vi "Create Queues for Logging and Transmission.vi"(8 "error in (no error)":errorcluster caption="错误输入（无错误）") -> (0 "error out":errorcluster caption="错误输出", 3 "Queues for Logging and Transmission":T1 caption="至记录与传输循环的队列")   [LabVIEW 2013]
doc: "本VI用于创建应用程序所需的所有消息队列。如应用程序需要两个以上消息队列，可右键单击上面的“消息队列”常量并选择“打开自定义类型”，将新的消息队列添加至该自定义类型，然后通过本VI进行初始化。"
uses:
  Queues for Logging and Transmission.ctl
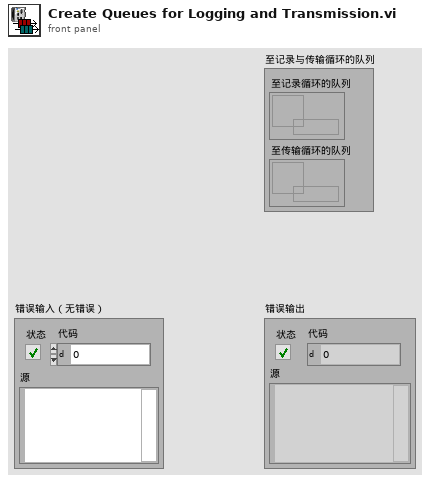
[diagram p1: front panel]
types:
  T1 = typedef "Queues for Logging and Transmission.ctl" = cluster{"Queue to Logging Loop":refnum<queue>, "Queue to Transmission Loop":refnum<queue>}
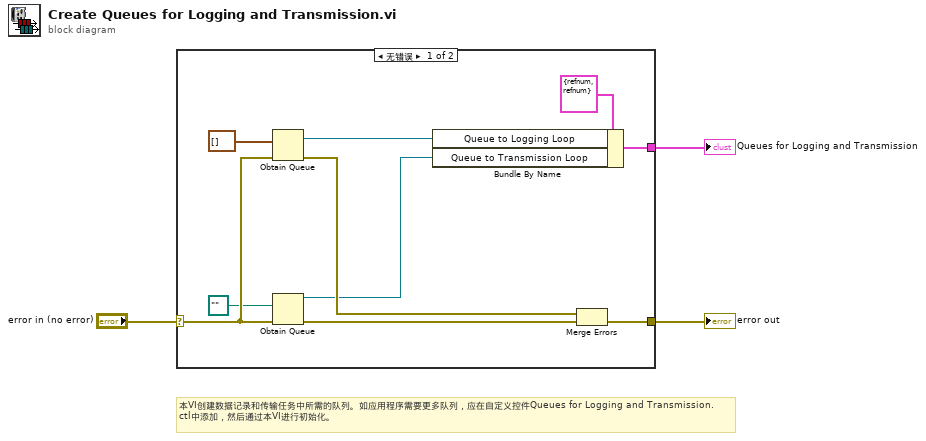
[diagram p0: block diagram]
diagram:
  # "本VI创建数据记录和传输任务中所需的队列。如应用程序需要更多队列，应在自定义控件Queues for Logging and Transmission.ctl中添加，然后通过本VI进行初始化。"
  n1 = case shown="无错误" "error in (no error)" {
    selector: "error in (no error)" -> [w10 w14]
    tunnel: [w12 w14] -> w3
    tunnel: [w13 _] -> w1
    frame No Error {
      n2 = Obtain Queue(element data type=waveform(dbl)[] [], error in (no error)=w10) -> (queue out=w6:refnum<queue>, error out=w9:errorcluster)  [unwired: 3 in, 1 out]
      n3 = Obtain Queue(element data type=path "", error in (no error)=w10) -> (queue out=w5:refnum<queue>, error out=w11:errorcluster)  [unwired: 3 in, 1 out]
      n4 = Bundle By Name(cluster=T1 {"Queue to Logging Loop"=refnum, "Queue to Transmission Loop"=refnum} ("Queues for Logging and Transmission"), "Queue to Logging Loop"=w6, "Queue to Transmission Loop"=w5) -> (w13:T1)
      n5 = Merge Errors(w9, w11) -> (w12:errorcluster)
    }
    frame Error {
    }
  }
  "error out" <- w3
  "Queues for Logging and Transmission" <- w1
